vi "ADCok.vi"(3 "PedOK":bool, 4 "Array":dbl[](array[numeric]), 5 "Vmax-1/2":dbl) -> (0 "Vmin":dbl, 1 "ADC voltages OK":bool=TRUE, 2 "Allok":bool)   [LabVIEW 2018]
panel:
  # "Checks ADC Voltages in range"
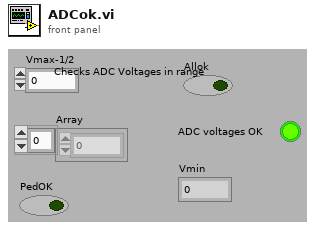
[diagram p1: front panel]
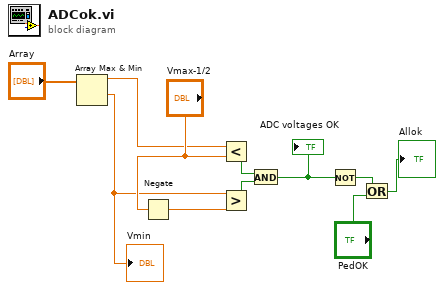
[diagram p0: block diagram]
diagram:
  n1 = Array Max & Min(array="Array") -> (max value=w6:dbl, min value=w1:dbl)  [unwired: 2 out]
  "Vmin" <- w1
  n2 = Negate(x="Vmax-1/2") -> (-x=w2:dbl)
  n3 = Less?(x=w6, y="Vmax-1/2") -> (x < y?=w4:bool)
  n4 = Greater?(x=w1, y=w2) -> (0:w3:bool)
  n5 = And(x=w4, y=w3) -> (x .and. y?=w8:bool)
  "ADC voltages OK" <- w8
  n6 = Not(x=w8) -> (.not. x?=w9:bool)
  n7 = Or(x=w9, y="PedOK") -> (x .or. y?=→"Allok":bool)
